vi "PH_gentec_M-Link.set current Settings to GUI.vi"(0 "i ref in":refnum<vi>, 5 "error in":errorcluster) -> (14 "i ref out":refnum<vi>, 19 "error out":errorcluster)   [LabVIEW 2014, in "PH_gentec_M-Link.lvlib"]
doc: "This VI indicates the current Settings at all relevant GUI elements."
uses:
  PH_gentec_M-Link.lvlib
  instr.lib/Gentec-M-Link/Driver/Type Defs/gentec-M-Link.Trigger Source.ctl
  PH_Basics/PH_Common/PH_Common.lvlib
  instr.lib/Gentec-M-Link/gentec-M-Link - Driver.lvlib
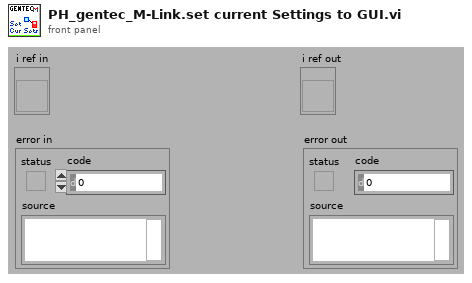
[diagram p1: front panel]
types:
  T1 = typedef "gentec-M-Link - Driver.lvlib/gentec-M-Link.Trigger Source.ctl" = u16
  T2 = typedef "PH_gentec_M-Link.lvlib/PH_gentec_M-Link.i attribute.ctl" = cluster{"GUI References":cluster{"Wanted Head Settings":refnum<vi>, "Current Head Settings":refnum<vi>, "Set Auto Range":refnum<vi>, "Trigger Polarity":refnum<vi>, "Trigger Source":refnum<vi>, "Waveform Averages":refnum<vi>, "Continuous":refnum<vi>, "get one Value":refnum<vi>}, "Wanted Head Settings":T3, "Current Head Settings":T3}
  T3 = typedef "PH_gentec_M-Link.lvlib/PH_gentec_M-Link.Head Settings.ctl" = cluster{"Measurement Mode":T4, "Enable Anticipation":bool, "Set Auto Range":bool, "Block Signal":bool, "Set Head Attenuator":bool, "Enable SSE":bool, "Trigger Polarity":T5, "Trigger Source":T1, "Waveform Averages":T6, "Set Zero":i32, "Current":i32, "Start Data Flow":bool}
  T4 = typedef "gentec-M-Link - Driver.lvlib/gentec-M-Link.Measurement Mode.ctl" = u16
  T5 = typedef "gentec-M-Link - Driver.lvlib/gentec-M-Link.Trigger Polarity.ctl" = u16
  T6 = typedef "gentec-M-Link - Driver.lvlib/gentec-M-Link.Waveform Averages.ctl" = u16
  T7 = enum8{"Enabled", "Disabled", "Disabled and Grayed Out"}
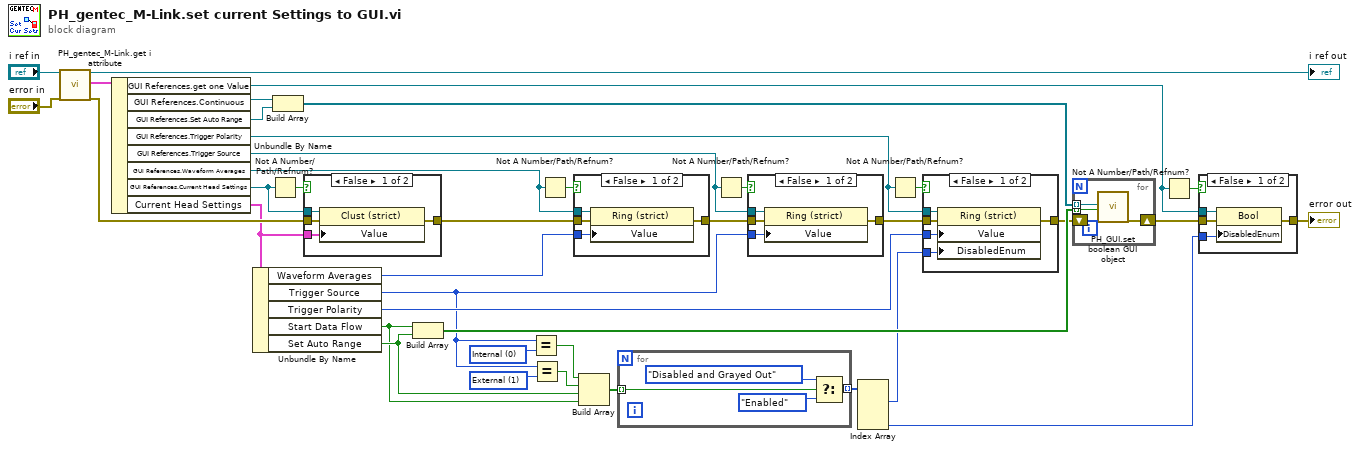
[diagram p0: block diagram]
diagram:
  w12 = T1 0 items=["Internal", "External"] ("Trigger Source")
  w13 = T1 1 items=["Internal", "External"] ("Trigger Source")
  n1 = call "PH_gentec_M-Link.get i attribute.vi"("i ref in"="i ref in", "error in (no error)"="error in") -> ("i ref out"=→"i ref out":refnum<vi>, "i attribute"=w39:T2, "error out"=w35:errorcluster)  [unwired: 15 in]
  n2 = Unbundle By Name(w39) -> ("GUI References.get one Value"=w14:refnum<vi>, "GUI References.Continuous"=w30:refnum<vi>, "GUI References.Set Auto Range"=w29:refnum<vi>, "GUI References.Trigger Polarity"=w20:refnum<vi>, "GUI References.Trigger Source"=w19:refnum<vi>, "GUI References.Waveform Averages"=w18:refnum<vi>, "GUI References.Current Head Settings"=w33:refnum<vi>, "Current Head Settings"=w32:T3)
  n3 = Unbundle By Name(w32) -> ("Waveform Averages"=w26:T6, "Trigger Source"=w10:T1, "Trigger Polarity"=w21:T5, "Start Data Flow"=w4:bool, "Set Auto Range"=w5:bool)
  n4 = Not A Number/Path/Refnum?(number/path/refnum=w33) -> (NaN/Path/Refnum?=w34:bool)
  n5 = Build Array(w30, w29) -> (w28:refnum<vi>[])
  n6 = case shown="False" w34 {
    tunnel: [w43 w44] -> w2
    tunnel: w33 -> [w42 _]
    tunnel: w35 -> [w41 w44]
    tunnel: w32 -> [w40 _]
    frame False {
      n7 = property class="Clust (strict)"(reference=w42, error in=w41, "Value"=w40) -> (error out=w43:errorcluster)  [unwired: 1 out]
    }
    frame True {
    }
  }
  n8 = Build Array(w4, w5) -> (w31:bool[])
  n9 = Equal?(x=w10, y=w12) -> (x = y?=w11:bool)
  n10 = Equal?(x=w10, y=w13) -> (x = y?=w6:bool)
  n11 = Not A Number/Path/Refnum?(number/path/refnum=w18) -> (NaN/Path/Refnum?=w27:bool)
  n12 = case shown="False" w27 {
    tunnel: [w48 w49] -> w24
    tunnel: w18 -> [w47 _]
    tunnel: w2 -> [w46 w49]
    tunnel: w26 -> [w45 _]
    frame False {
      n13 = property class="Ring (strict)"(reference=w47, error in=w46, "Value"=w45) -> (error out=w48:errorcluster)  [unwired: 1 out]
    }
    frame True {
    }
  }
  n14 = Build Array(w11, w6, w5, w4) -> (w7:bool[])
  n15 = for {
    tunnel: w7 -> [w51] mode=indexing
    tunnel: [w50] -> w9 mode=indexing
    n16 = Select(t=T7."Disabled and Grayed Out" ("Disabled"), s=w51, f=T7."Enabled" ("Disabled")) -> (s? t:f=w50:T7)
  }
  n17 = Not A Number/Path/Refnum?(number/path/refnum=w19) -> (NaN/Path/Refnum?=w25:bool)
  n18 = case shown="False" w25 {
    tunnel: [w57 w58] -> w22
    tunnel: w19 -> [w56 _]
    tunnel: w24 -> [w55 w58]
    tunnel: w10 -> [w54 _]
    frame False {
      n19 = property class="Ring (strict)"(reference=w56, error in=w55, "Value"=w54) -> (error out=w57:errorcluster)  [unwired: 1 out]
    }
    frame True {
    }
  }
  n20 = Index Array(array=w9) -> (element #1=w8:T7, element #4=w3:T7)  [unwired: 4 in, 2 out]
  n21 = Not A Number/Path/Refnum?(number/path/refnum=w20) -> (NaN/Path/Refnum?=w23:bool)
  n22 = case shown="False" w23 {
    tunnel: [w63 w64] -> w1
    tunnel: w20 -> [w62 _]
    tunnel: w22 -> [w61 w64]
    tunnel: w21 -> [w60 _]
    tunnel: w8 -> [w59 _]
    frame False {
      n23 = property class="Ring (strict)"(reference=w62, error in=w61, "Value"=w60, "DisabledEnum"=w59) -> (error out=w63:errorcluster)  [unwired: 1 out]
    }
    frame True {
    }
  }
  n24 = for {
    tunnel: w31 -> [w66] mode=indexing
    shift-right: [w67] -> w17
    shift-left: w1 -> [w68]
    tunnel: w28 -> [w65] mode=indexing
    n25 = call "PH_GUI.set boolean GUI object.vi"("Boolean Knob GUI Ref"=w65, "Value"=w66, "error in (no error)"=w68) -> ("error out"=w67:errorcluster)  [unwired: 16 in]
  }
  n26 = Not A Number/Path/Refnum?(number/path/refnum=w14) -> (NaN/Path/Refnum?=w15:bool)
  n27 = case shown="False" w15 {
    tunnel: [w72 w73] -> w16
    tunnel: w14 -> [w71 _]
    tunnel: w17 -> [w70 w73]
    tunnel: w3 -> [w69 _]
    frame False {
      n28 = property class="Bool"(reference=w71, error in=w70, "DisabledEnum"=w69) -> (error out=w72:errorcluster)  [unwired: 1 out]
    }
    frame True {
    }
  }
  "error out" <- w16
